vi "Init.vi"(8 "error in (no error)":errorcluster, 11 "bt_Blackboard in":refnum<class "bt_Blackboard.lvclass">) -> (0 "error out":errorcluster, 3 "bt_Blackboard out":refnum<class "bt_Blackboard.lvclass">)   [LabVIEW 2021, in "BT.lvlib" / "bt_Blackboard.lvclass"]
uses:
  bt_Blackboard.lvclass
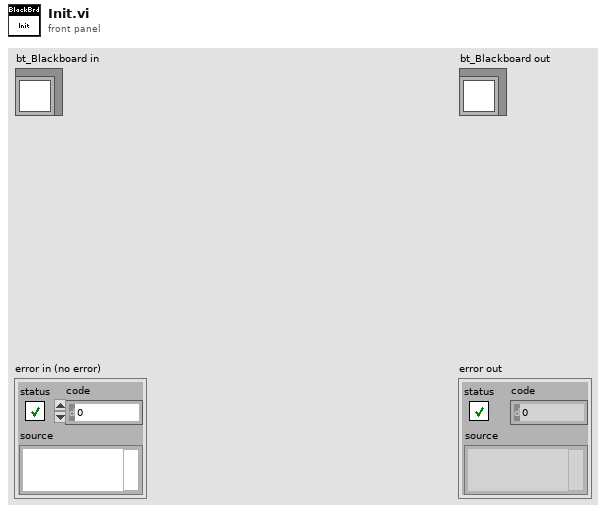
[diagram p1: front panel]
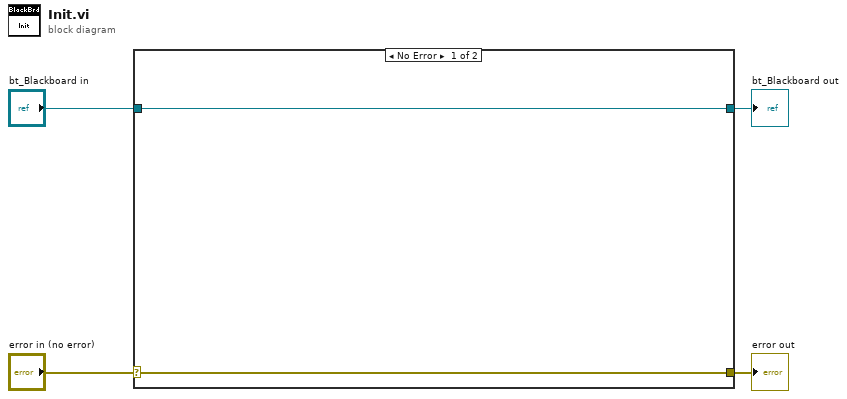
[diagram p0: block diagram]
diagram:
  n1 = case shown="No Error" "error in (no error)" {
    selector: "error in (no error)" -> [w5 w8]
    tunnel: [w5 w8] -> w3
    tunnel: [w6 w7] -> w1
    tunnel: "bt_Blackboard in" -> [w6 w7]
    frame No Error {
    }
    frame Error {
    }
  }
  "error out" <- w3
  "bt_Blackboard out" <- w1
